vi "Homework #7.vi"() -> ()   [LabVIEW 2017]
uses:
  Main Global.vi
panel:
  out "String Results":string
  in  "stop":bool
  out "Results":cluster{"Results":dbl[], "Done":bool}
  in  "Calculate":bool
  in  "Numeric #2":dbl
  in  "Numeric #1":dbl
  in  "Calculations":T1(array[ring])
  # "This is a modification!"
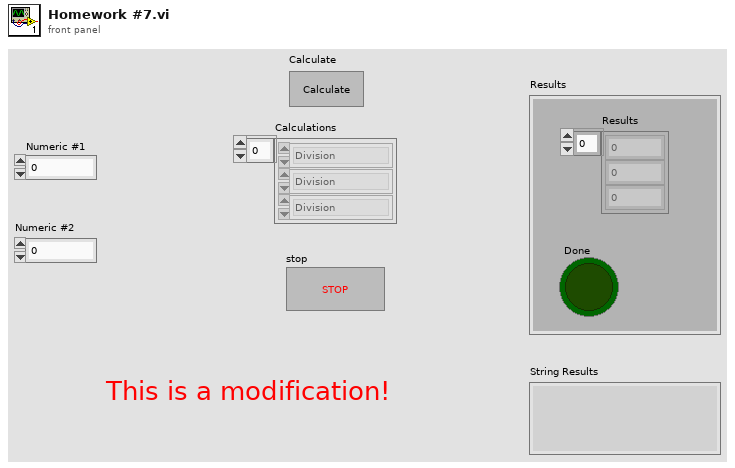
[diagram p1: front panel]
types:
  T1 = enum16{"Division", "Multiplication", "Subtraction"}[]
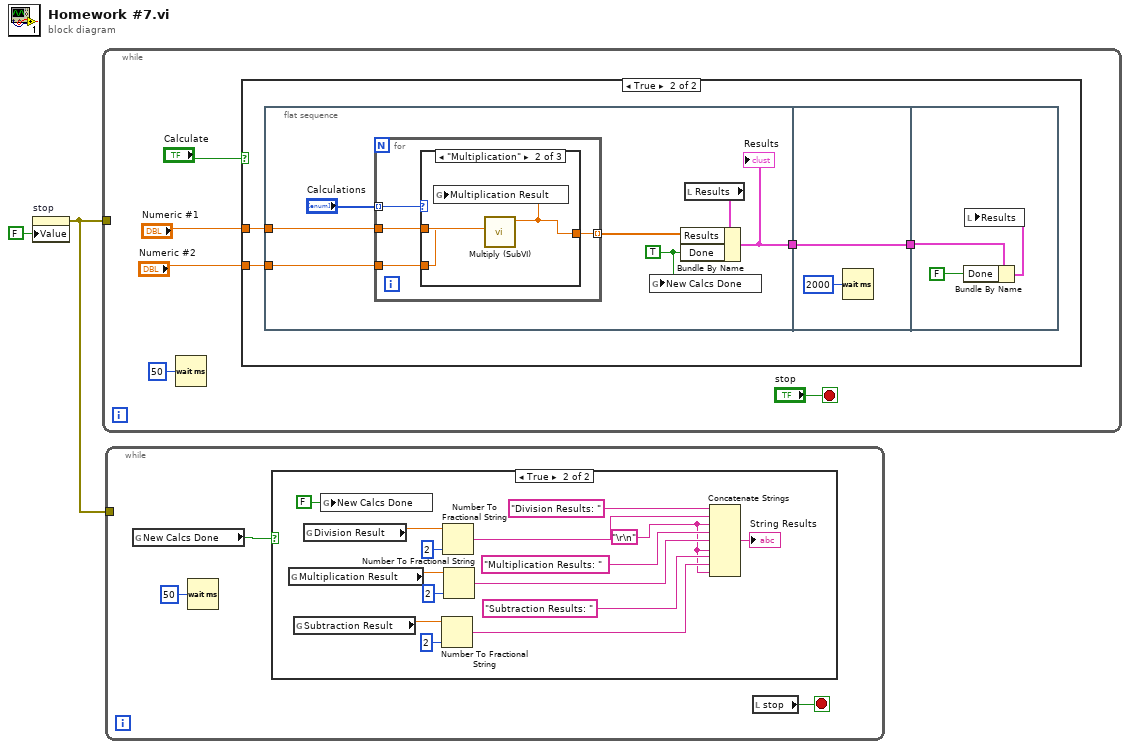
[diagram p0: block diagram]
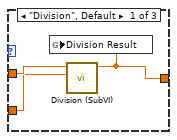
[diagram p4: hidden frame]
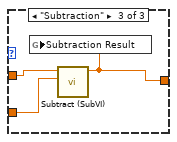
[diagram p5: hidden frame]
diagram:
  n1 = property on="stop" class="Bool (strict)"("Value"=FALSE ("stop")) -> (error out=w1:errorcluster)  [unwired: 2 in, 1 out]
  n2 = while {
    tunnel: w1 -> [_]
    stop <- "stop" stop-if-true
    n3 = Wait (ms)(milliseconds to wait=u32 50) -> ()  [unwired: 1 out]
    n4 = case shown="True" "Calculate" {
      tunnel: "Numeric #1" -> [_ w11]
      tunnel: "Numeric #2" -> [_ w10]
      frame False {
      }
      frame True {
        n5 = flat-sequence {
          tunnel: [w13] -> w8
          tunnel: w10 -> [w16]
          tunnel: w11 -> [w17]
          tunnel: [w32] -> w9
          tunnel: w8 -> [w32]
          tunnel: w9 -> [w36]
          frame #0 {
            w12 = TRUE ("Done")
            n6 = for {
              tunnel: "Calculations" -> [w22] mode=indexing
              tunnel: w17 -> [w21]
              tunnel: w16 -> [w20]
              tunnel: [w19] -> w14 mode=indexing
              n7 = case shown="\"Multiplication\"" w22 {
                tunnel: w21 -> [w25 w28 w31]
                tunnel: w20 -> [w24 w27 w30]
                tunnel: [w23 w26 w29] -> w19
                frame "Division", Default {
                  n8 = call "Division (SubVI).vi"("Numeric #2"=w24, "Numeric #1"=w25) -> ("Numeric"=w23:dbl)  [unwired: 9 in]
                  n9 = global write "Main Global.vi" "Division Result"(w23) -> ()
                }
                frame "Multiplication" {
                  n10 = call "Multiply (SubVI).vi"("Numeric #2"=w27, "Numeric #1"=w28) -> ("Numeric"=w26:dbl)  [unwired: 9 in]
                  n11 = global write "Main Global.vi" "Multiplication Result"(w26) -> ()
                }
                frame "Subtraction" {
                  n12 = call "Subtract (SubVI).vi"("Numeric #2"=w30, "Numeric #1"=w31) -> ("Numeric"=w29:dbl)  [unwired: 9 in]
                  n13 = global write "Main Global.vi" "Subtraction Result"(w29) -> ()
                }
              }
            }
            n14 = global write "Main Global.vi" "New Calcs Done"(w12) -> ()
            n15 = local read "Results"() -> (w15:cluster{"Results":dbl[], "Done":bool})
            n16 = Bundle By Name(cluster=w15, "Results"=w14, "Done"=w12) -> (w13:cluster{"Results":dbl[], "Done":bool})
            "Results" <- w13
          }
          frame #1 {
            n17 = Wait (ms)(milliseconds to wait=u32 2000) -> ()  [unwired: 1 out]
          }
          frame #2 {
            n18 = Bundle By Name(cluster=w36, "Done"=FALSE) -> (w35:cluster{"Results":dbl[], "Done":bool})
            n19 = local write "Results"(w35) -> ()
          }
        }
      }
    }
  }
  n20 = while {
    tunnel: w1 -> [_]
    stop <- w39 stop-if-true
    n21 = global read "Main Global.vi" "New Calcs Done"() -> (w38:bool)
    n22 = Wait (ms)(milliseconds to wait=u32 50) -> ()  [unwired: 1 out]
    n23 = case shown="True" w38 {
      frame False {
      }
      frame True {
        w42 = "\r\n"
        n24 = global read "Main Global.vi" "Multiplication Result"() -> (w51:dbl)
        n25 = global read "Main Global.vi" "Subtraction Result"() -> (w50:dbl)
        n26 = global read "Main Global.vi" "Division Result"() -> (w54:dbl)
        n27 = global write "Main Global.vi" "New Calcs Done"(FALSE ("New Calcs Done")) -> ()
        n28 = Number To Fractional String(number=w50, precision (6)=i16 2) -> (F-format string=w43:string)  [unwired: 2 in]
        n29 = Number To Fractional String(number=w54, precision (6)=i16 2) -> (F-format string=w47:string)  [unwired: 2 in]
        n30 = Number To Fractional String(number=w51, precision (6)=i16 2) -> (F-format string=w45:string)  [unwired: 2 in]
        n31 = Concatenate Strings("Division Results: ", w47, w42, "Multiplication Results: ", w45, w42, "Subtraction Results: ", w43, w42) -> (→"String Results":string)
      }
    }
    n32 = local read "stop"() -> (w39:bool)
  }
